vi "Producer consumer coke machine NIVerified.vi"() -> ()   [LabVIEW 2016]
uses:
  Coke Machine State Control.ctl
panel:
  out "Current State":T1=enum."Wait"
  in  "Quarter":bool
  out "Change Return":string="0 Cents"
  in  "Coke Display":u16(ring)
  in  "Nickel":bool
  in  "Return":bool
  in  "Dime":bool
  out "Deposited":i32
  # "Overview: This VI uses the Producer/Consumer design pattern to emulate the behavior of a vending machine.\nRequirements: LabVIEW 2012 (or compatible)\nInstructions: Load and run this VI in LabVIEW."
  # "50 Cents"
  # "50 Cents"
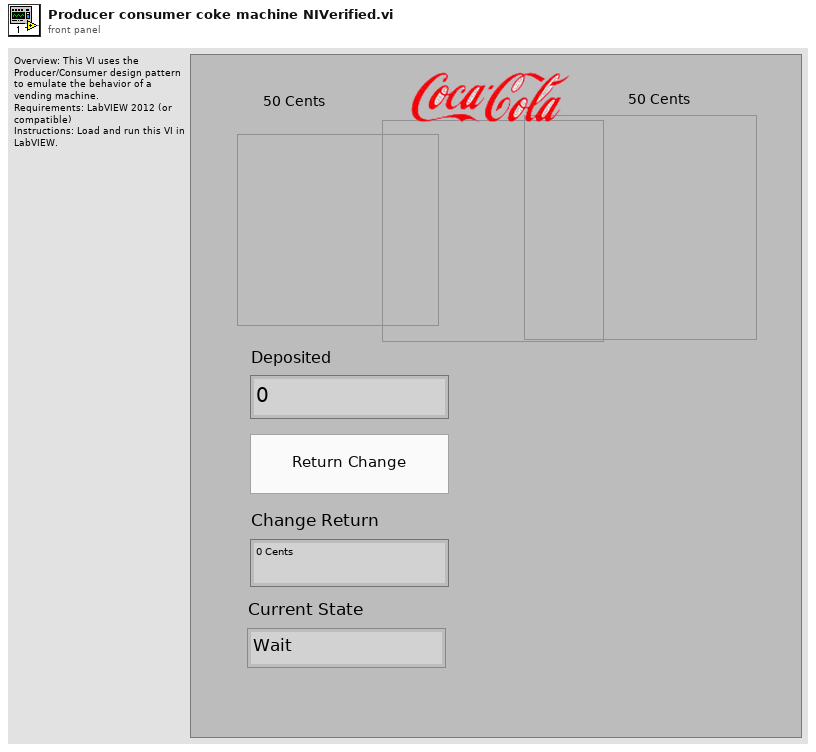
[diagram p1: front panel]
types:
  T1 = typedef "Coke Machine State Control.ctl" = enum16{"Initialize", "Wait", "Nickel", "Dime", "Quarter", "Vend", "Change", "Exit"}
  T2 = enum16{"Initialize", "Wait", "Nickel", "Dime", "Quarter", "Vend", "Change", "Exit"}
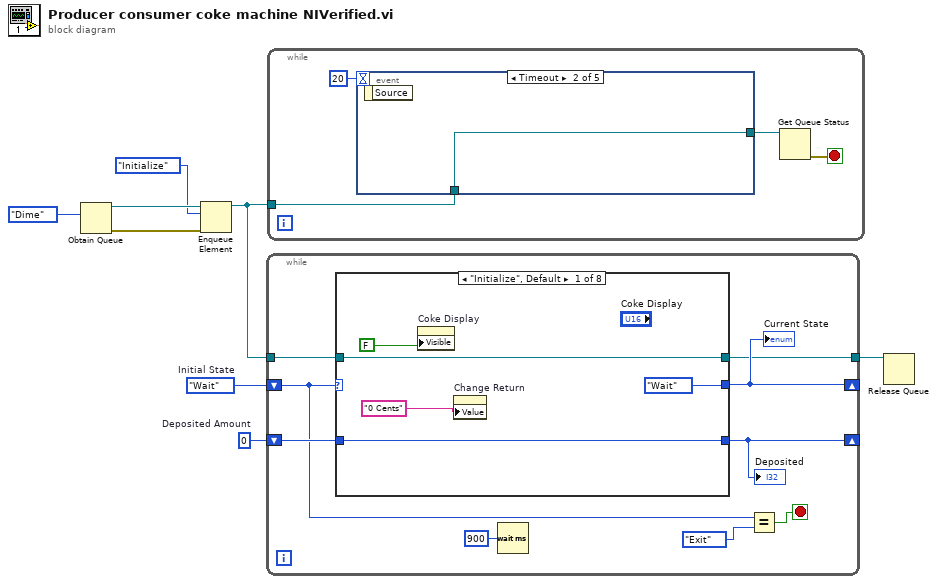
[diagram p0: block diagram]
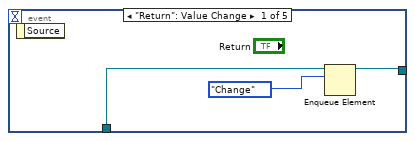
[diagram p2: hidden frame]
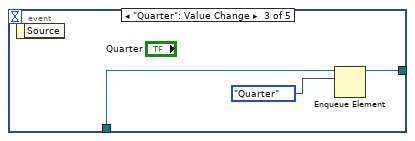
[diagram p3: hidden frame]
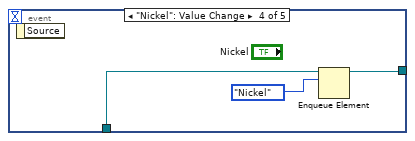
[diagram p4: hidden frame]
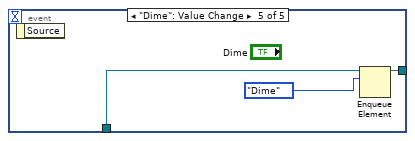
[diagram p5: hidden frame]
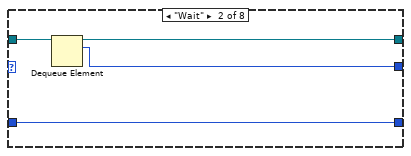
[diagram p6: hidden frame]
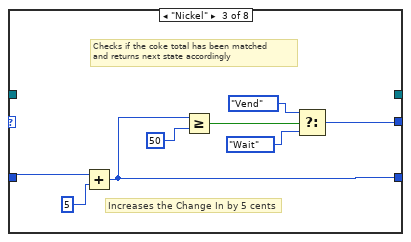
[diagram p7: hidden frame]
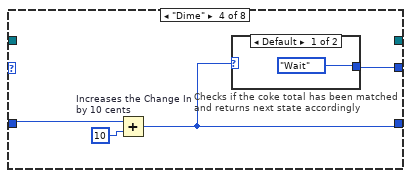
[diagram p8: hidden frame]
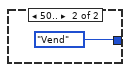
[diagram p9: hidden frame]
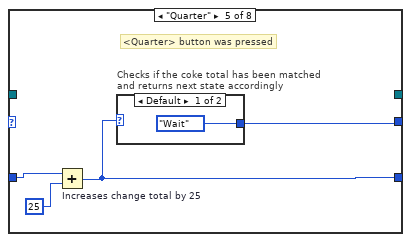
[diagram p10: hidden frame]
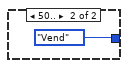
[diagram p11: hidden frame]
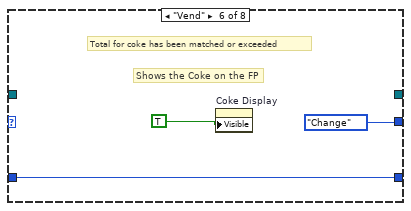
[diagram p12: hidden frame]
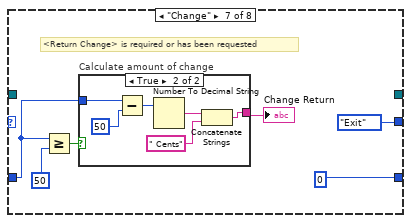
[diagram p13: hidden frame]
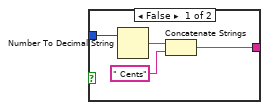
[diagram p14: hidden frame]
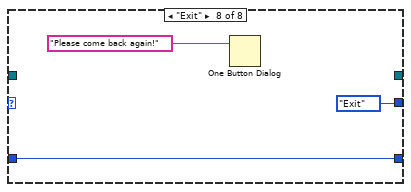
[diagram p15: hidden frame]
diagram:
  w7 = Coke_Machine_State_Control."Wait"  # Initial State
  w8 = 0  # Deposited Amount
  n1 = Obtain Queue(element data type=Coke_Machine_State_Control."Dime" ("Initial State")) -> (queue out=w6:refnum<queue>, error out=w4:errorcluster)  [unwired: 3 in, 2 out]
  n2 = Enqueue Element(queue=w6, element=Coke_Machine_State_Control."Initialize" ("Initial State"), error in (no error)=w4) -> (queue out=w5:refnum<queue>)  [unwired: 3 out]
  n3 = while {
    shift-right: [w12] -> _
    shift-left: w7 -> [w9]
    shift-right: [w13] -> _
    shift-left: w8 -> [w16]
    tunnel: w5 -> [w10]
    tunnel: [w10] -> w3
    stop <- w15 stop-if-true
    n4 = case shown="\"Initialize\", Default" w9 {
      tunnel: [w20 w24 w29 w35 w41 w47 0 w65] -> w13
      tunnel: w16 -> [w20 w24 w31 w34 w40 w47 w50 w65]
      tunnel: w10 -> [_ w23 _ _ _ _ _ _]
      tunnel: [_ w22 _ _ _ _ _ _] -> _
      tunnel: [Coke_Machine_State_Control."Wait" ("Initial State") w21 w25 w33 w39 Coke_Machine_State_Control."Change" ("Initial State") Coke_Machine_State_Control."Exit" ("Initial State") Coke_Machine_State_Control."Exit" ("Initial State")] -> w12
      frame "Initialize", Default {
        n5 = property on="Coke Display" class="Ring (strict)"("Visible"=FALSE) -> ()  [unwired: 2 in, 2 out]
        n6 = property on="Change Return" class="Str"("Value"="0 Cents" ("Change")) -> ()  [unwired: 2 in, 2 out]
      }
      frame "Wait" {
        n7 = Dequeue Element(queue=w23) -> (queue out=w22:refnum<queue>, element=w21:T1)  [unwired: 1 in, 3 out]
      }
      frame "Nickel" {
        # "Increases the Change In by 5 cents"
        # "Checks if the coke total has been matched\nand returns next state accordingly"
        n8 = Add(x=w31, y=5) -> (x+y=w29:i32)
        n9 = Greater Or Equal?(x=w29, y=50) -> (x >= y?=w30:bool)
        n10 = Select(t=Coke_Machine_State_Control."Vend" ("Initial State"), s=w30, f=Coke_Machine_State_Control."Wait" ("Initial State")) -> (s? t:f=w25:T1)
      }
      frame "Dime" {
        n11 = Add "Increases the Change In by 10 cents"(x=w34, y=10) -> (x+y=w35:i32)
        n12 = case "Checks if the coke total has been matched\nand returns next state accordingly" shown="Default" w35 {
          tunnel: [Coke_Machine_State_Control."Wait" ("Initial State") Coke_Machine_State_Control."Vend" ("Initial State")] -> w33
          frame Default {
          }
          frame 50.. {
          }
        }
      }
      frame "Quarter" {
        # "<Quarter> button was pressed"
        n13 = Add "Increases change total by 25"(x=w40, y=25) -> (x+y=w41:i32)
        n14 = case "Checks if the coke total has been matched\nand returns next state accordingly" shown="Default" w41 {
          tunnel: [Coke_Machine_State_Control."Wait" ("Initial State") Coke_Machine_State_Control."Vend" ("Initial State")] -> w39
          frame Default {
          }
          frame 50.. {
          }
        }
      }
      frame "Vend" {
        # "Total for coke has been matched or exceeded"
        # "Shows the Coke on the FP"
        n15 = property on="Coke Display" class="Ring (strict)"("Visible"=TRUE) -> ()  [unwired: 2 in, 2 out]
      }
      frame "Change" {
        # "<Return Change> is required or has been requested"
        n16 = Greater Or Equal?(x=w50, y=50) -> (x >= y?=w51:bool)
        n17 = case "Calculate amount of change" shown="True" w51 {
          tunnel: [w55 w61] -> w49
          tunnel: w50 -> [w54 w59]
          frame False {
            n18 = Number To Decimal String(number=w54) -> (decimal integer string=w57:string)  [unwired: 1 out]
            n19 = Concatenate Strings(w57, " Cents" ("string")) -> (w55:string)
          }
          frame True {
            n20 = Subtract(x=w59, y=50 ("x")) -> (x-y=w60:i32)
            n21 = Number To Decimal String(number=w60) -> (decimal integer string=w63:string)  [unwired: 1 out]
            n22 = Concatenate Strings(w63, " Cents" ("string")) -> (w61:string)
          }
        }
        "Change Return" <- w49
      }
      frame "Exit" {
        n23 = One Button Dialog(message="Please come back again!") -> ()  [unwired: 2 out]
      }
    }
    "Deposited" <- w13
    "Current State" <- w12
    n24 = Wait (ms)(milliseconds to wait=u32 900 ("millisecond multiple")) -> ()  [unwired: 1 out]
    n25 = Equal?(x=w9, y=Coke_Machine_State_Control."Exit" ("Initial State")) -> (x = y?=w15:bool)
  }
  n26 = while {
    tunnel: w5 -> [w69]
    stop <- w67 stop-if-true
    n27 = event shown="[1] Timeout" {
      selector: _ -> [_ _ _ _ _]
      dyn-events: _ -> [_ _ _ _ _]
      timeout: 20 -> [_ _ _ _ _]
      tunnel: w69 -> [w73 w74 w76 w79 w82]
      tunnel: [w72 w74 w77 w80 w81] -> w68
      event "Return": Value Change {
        n28 = event-data() -> ()  [unwired: 2 out]
        n29 = Enqueue Element(queue=w73, element=Coke_Machine_State_Control."Change" ("Initial State")) -> (queue out=w72:refnum<queue>)  [unwired: 1 in, 3 out]
      }
      event Timeout {
        n30 = event-data() -> ()  [unwired: 2 out]
      }
      event "Quarter": Value Change {
        n31 = event-data() -> ()  [unwired: 2 out]
        n32 = Enqueue Element(queue=w76, element=Coke_Machine_State_Control."Quarter" ("Initial State")) -> (queue out=w77:refnum<queue>)  [unwired: 1 in, 3 out]
      }
      event "Nickel": Value Change {
        n33 = event-data() -> ()  [unwired: 2 out]
        n34 = Enqueue Element(queue=w79, element=Coke_Machine_State_Control."Nickel" ("Initial State")) -> (queue out=w80:refnum<queue>)  [unwired: 1 in, 3 out]
      }
      event "Dime": Value Change {
        n35 = event-data() -> ()  [unwired: 2 out]
        n36 = Enqueue Element(queue=w82, element=T2."Dime" ("Enum")) -> (queue out=w81:refnum<queue>)  [unwired: 1 in, 3 out]
      }
    }
    n37 = Get Queue Status(queue=w68) -> (error out=w67:errorcluster)  [unwired: 1 in, 8 out]
  }
  n38 = Release Queue(queue=w3) -> ()  [unwired: 1 in, 4 out]
